vi "I32Notifier Send.vi"(8 "error in (no error)":errorcluster, 10 "element":i32, 11 "I32Notifier in":refnum<class "I32Notifier.lvclass">) -> (0 "error out":errorcluster, 1 "timed out?":bool, 3 "I32Notifier out":refnum<class "I32Notifier.lvclass">)   [LabVIEW 2018, in "I32Notifier.lvclass"]
uses:
  I32Notifier.lvclass
  I32Notifier.lvclass/I32Notifier.ctl
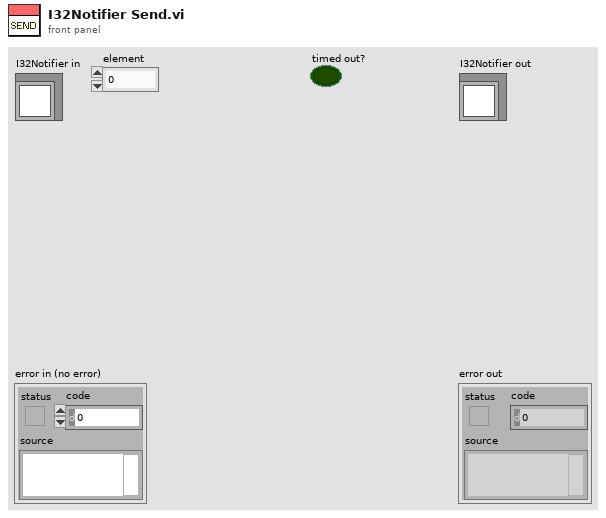
[diagram p1: front panel]
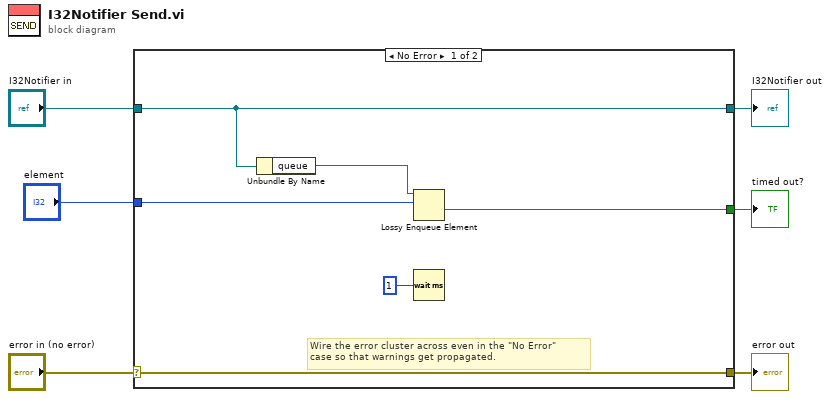
[diagram p0: block diagram]
diagram:
  n1 = case shown="No Error" "error in (no error)" {
    selector: "error in (no error)" -> [w12 w14]
    tunnel: [w12 w14] -> w5
    tunnel: [w11 w13] -> w3
    tunnel: "I32Notifier in" -> [w11 w13]
    tunnel: "element" -> [w9 _]
    tunnel: [w8 _] -> w1
    frame No Error {
      # "Wire the error cluster across even in the \"No Error\"\ncase so that warnings get propagated."
      n2 = Unbundle By Name(w11) -> ("queue"=w10:refnum<queue>)
      n3 = Lossy Enqueue Element(queue=w10, element=w9) -> (overflow?=w8:bool)  [unwired: 1 in, 3 out]
      n4 = Wait (ms)(milliseconds to wait=u32 1) -> ()  [unwired: 1 out]
    }
    frame Error {
    }
  }
  "error out" <- w5
  "I32Notifier out" <- w3
  "timed out?" <- w1
